vi "InAs TED Characterise - PicoAmmeter plus temperature.vi"() -> ()   [LabVIEW 2024]
uses:
  <instrlib>/Keithley 648X Series/Keithley 648X Series.lvlib
panel:
  in  "stop":bool
  out "element":dbl
  in  "Tab Control":enum32{"Page 1", "Page 2"}(tab)
  out "InAs Detector Response":cluster{"Ramp Pattern":dbl[], dbl[]}(graph)
  out "Temperature Chart":dynamicdata(graph)
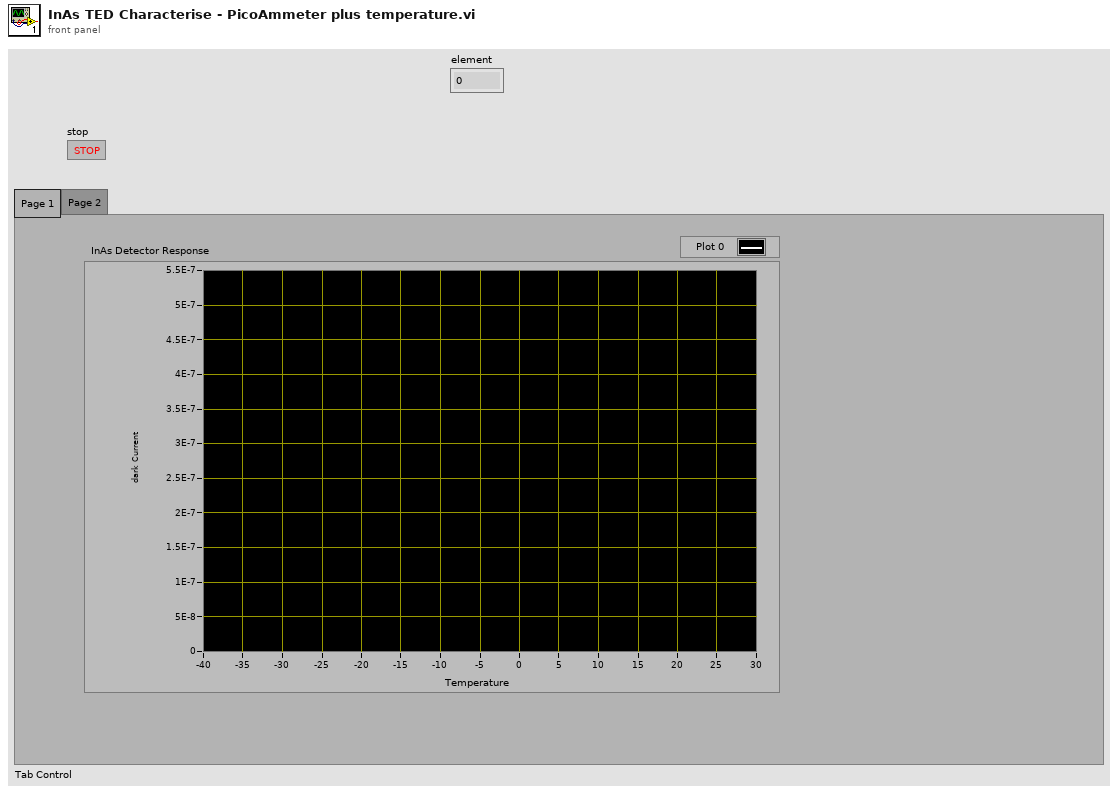
[diagram p1: front panel]
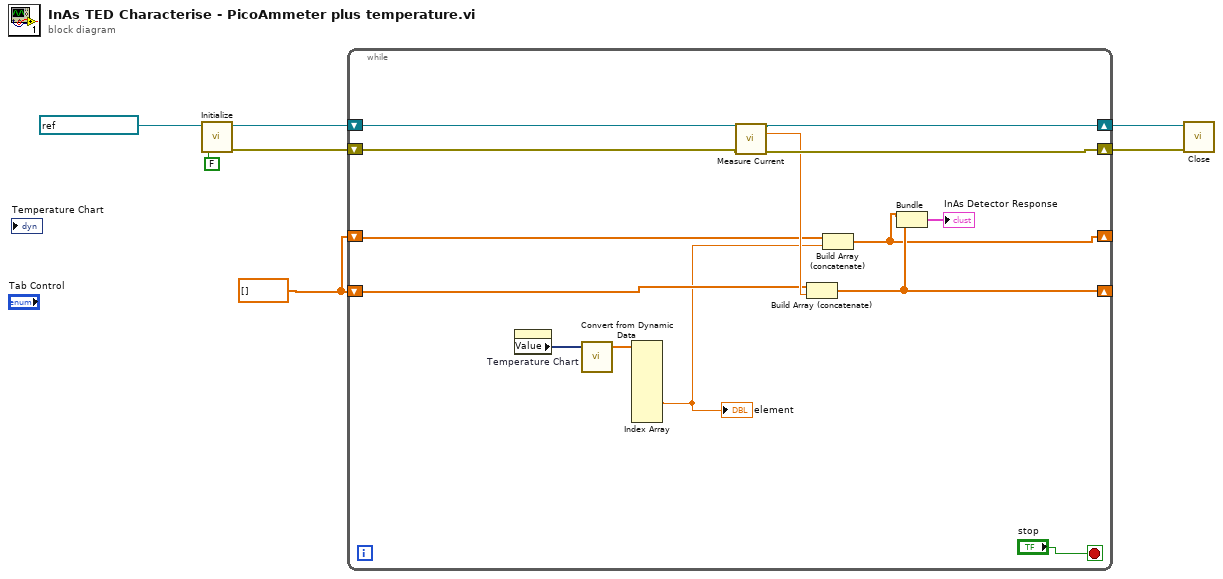
[diagram p0: block diagram]
diagram:
  w1 = dbl[] []
  n1 = call <instrlib>:"Initialize.vi"("ID Query (True)"=FALSE ("Reset (True)"), "VISA resource name"=refnum<visa-resource-name> "Picoammeter") -> ("error out"=w2:errorcluster, "VISA resource name out"=w3:refnum<visa-resource-name>)  [unwired: 8 in]
  n2 = while {
    shift-right: [w21] -> w6
    shift-left: w3 -> [w19]
    shift-right: [w20] -> w5
    shift-left: w2 -> [w18]
    shift-right: [w12] -> _
    shift-left: w1 -> [w13]
    shift-right: [w9] -> _
    shift-left: w1 -> [w11]
    stop <- "stop" stop-if-true
    n3 = property on="Temperature Chart" class="WFChart (strict)"() -> ("Value"=w15:dynamicdata)  [unwired: 2 in, 2 out]
    n4 = call "Convert from Dynamic Data"("Dynamic Data Type"=w15) -> ("Array"=w14:dbl[])  [unwired: 3 in]
    n5 = Index Array(array=w14) -> (element #6=w8:dbl)  [unwired: 8 in, 7 out]
    "element" <- w8
    n6 = call <instrlib>:"Measure Current.vi"("VISA resource name"=w19, "error in (no error)"=w18) -> ("VISA resource name out"=w21:refnum<visa-resource-name>, "Measurement"=w16:dbl, "error out"=w20:errorcluster)  [unwired: 11 in]
    n7 = Build Array (concatenate)(w13, w16) -> (w12:dbl[])
    n8 = Build Array (concatenate)(w11, w8) -> (w9:dbl[])
    n9 = Bundle(w9, w12) -> (→"InAs Detector Response":cluster{dbl[], dbl[]})  [unwired: 1 in]
  }
  n10 = call <instrlib>:"Close.vi"("error in (no error)"=w5, "VISA resource name"=w6) -> ()  [unwired: 9 in, 1 out]
